vi "set view class name.vi"(8 "error in":errorcluster, 10 "view class":string, 11 "configuration in":refnum<class "NISE_CEF_serializable configuration.lvclass">) -> (0 "error out":errorcluster, 3 "configuration out":refnum<class "NISE_CEF_serializable configuration.lvclass">)   [LabVIEW 2013, in "NISE_CEF_serializable configuration.lvclass"]
uses:
  NISE_CEF_serializable configuration.lvclass
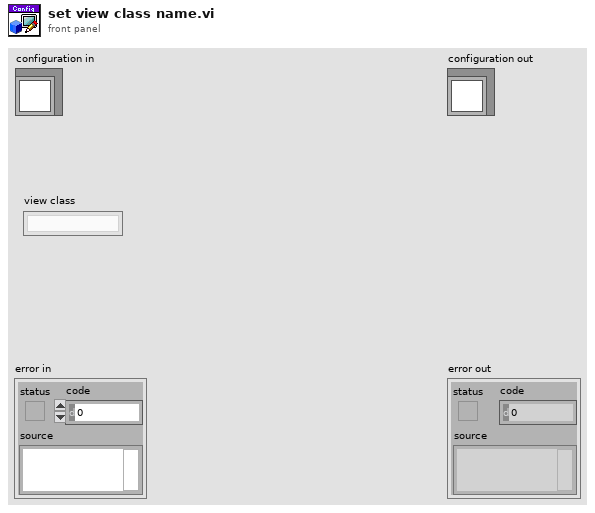
[diagram p1: front panel]
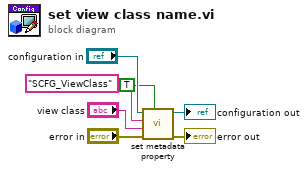
[diagram p0: block diagram]
diagram:
  n1 = call "set metadata property.vi"("overwrite?"=TRUE, "error in"="error in", "value"="view class", "key"="SCFG_ViewClass", "configuration in"="configuration in") -> ("error out"=→"error out":errorcluster, "configuration out"=→"configuration out":refnum<class "NISE_CEF_serializable configuration.lvclass">)  [unwired: 5 in]
